vi "Generate Digital Waveform in LV.vi"(0 "Size":i32=1000) -> (1 "Y":digitaldata, 2 "Digital Waveform array":digitalwaveform[](array[waveform]), 3 "digital waveform":digitalwaveform(waveform)={"t0"=timestamp(0 s since 1904-01-01), "dt"=0.0, "Y"={"transitions"=[], "data"=[]}, "error"={"status"=FALSE, "code"=37421928, "source"=""}}, 4 "compressed digital waveform":digitalwaveform(waveform)={"t0"=timestamp(0 s since 1904-01-01), "dt"=0.0, "Y"={"transitions"=[], "data"=[]}, "error"={"status"=FALSE, "code"=37421928, "source"=""}}, 5 "t0":timestamp, 6 "dt":dbl)   [LabVIEW 2013]
uses:
  <vilib>/Waveform/DWDTOps.llb/DWDT Boolean Array to Digital.vi
  <vilib>/Waveform/DWDTOps.llb/DWDT Compress Digital.vi
panel:
  out "Digital Waveform Graph":digitalwaveform(graph)
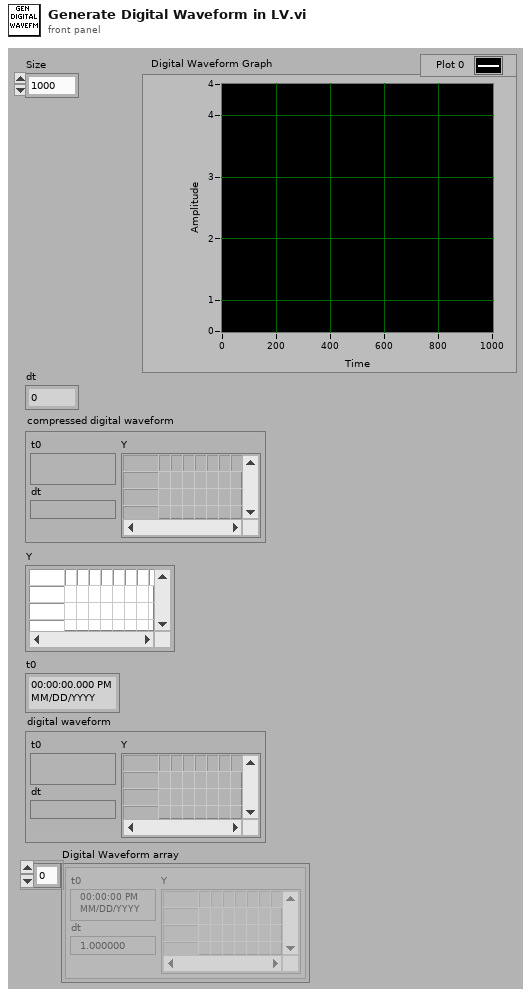
[diagram p1: front panel]
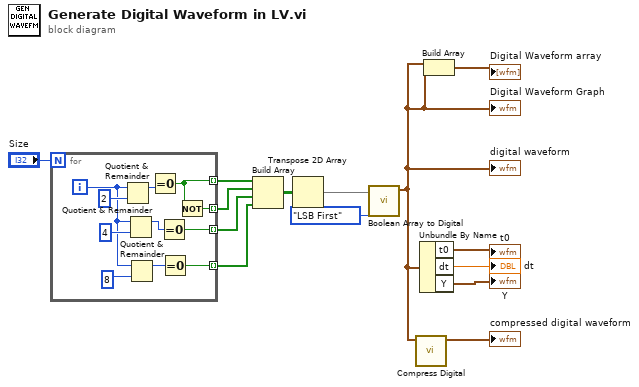
[diagram p0: block diagram]
diagram:
  n1 = for {
    N: "Size" -> [_]
    tunnel: [w23] -> w13 mode=indexing
    tunnel: [w22] -> w12 mode=indexing
    tunnel: [w20] -> w11 mode=indexing
    tunnel: [w15] -> w10 mode=indexing
    i -> [w18]
    n2 = Quotient & Remainder(x=w18, y=2) -> (x-y*floor(x/y)=w24:i32)  [unwired: 1 out]
    n3 = Quotient & Remainder(x=w18, y=4) -> (x-y*floor(x/y)=w21:i32)  [unwired: 1 out]
    n4 = Quotient & Remainder(x=w18, y=8) -> (x-y*floor(x/y)=w16:i32)  [unwired: 1 out]
    n5 = Equal To 0?(x=w24) -> (x = 0?=w23:bool)
    n6 = Equal To 0?(x=w21) -> (x = 0?=w20:bool)
    n7 = Equal To 0?(x=w16) -> (x = 0?=w15:bool)
    n8 = Not(x=w23) -> (.not. x?=w22:bool)
  }
  n9 = Build Array(w13, w12, w11, w10) -> (w9:bool[][])
  n10 = Transpose 2D Array(2D array=w9) -> (transposed array=w7:bool[][])
  n11 = call-poly <vilib>:"Boolean Array to Digital.vi"("mode"=enum16{"LSB First", "MSB First"}."LSB First", "boolean array"=w7) -> ("digital waveform"=w2:digitalwaveform)  [unwired: 3 in, 6 out]
  "Digital Waveform Graph" <- w2
  "digital waveform" <- w2
  n12 = call-poly <vilib>:"Compress Digital.vi"("uncompressed digital waveform"=w2) -> ("compressed digital waveform"=→"compressed digital waveform":digitalwaveform)  [unwired: 1 in, 9 out]
  n13 = Unbundle By Name(w2) -> ("t0"=→"t0":timestamp, "dt"=→"dt":dbl, "Y"=→"Y":digitaldata)
  n14 = Build Array(w2, w2) -> (→"Digital Waveform array":digitalwaveform[])
